vi "Read Sequential Addresses (CMD ONLY).vi"(7 "Target IC (1-8)":u8, 8 "error in (no error)":errorcluster, 9 "Addresses to Read":u16 format="%0.0f", 10 "Starting Address":u16 format="%04x", 11 "FPGA Interface in":refnum<class "FPGA Interface.lvclass">) -> (0 "error out":errorcluster)   [LabVIEW 2020, in "BCI-1553 API.lvlib" / "FPGA Interface.lvlib" / "FPGA Interface.lvclass"]
doc: "Reads a series of consecutive addresses from a component in the 1553 Session. Sequential addressing cannot be used on addresses from 0x0400 to 0x0800. This method does not block and will not wait for data to return from the specified component."
uses:
  FPGA Interface.lvclass
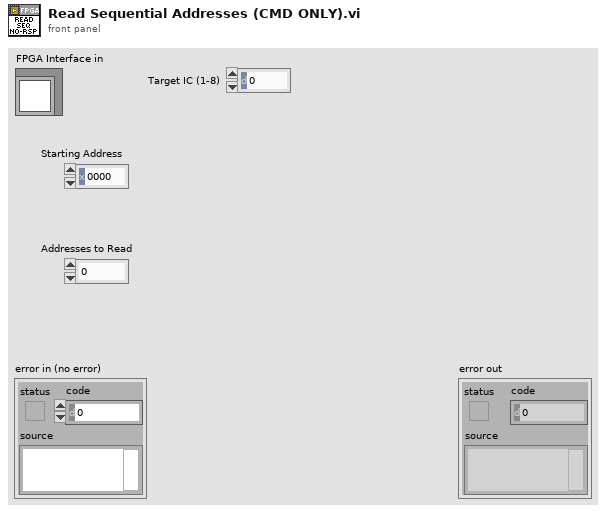
[diagram p1: front panel]
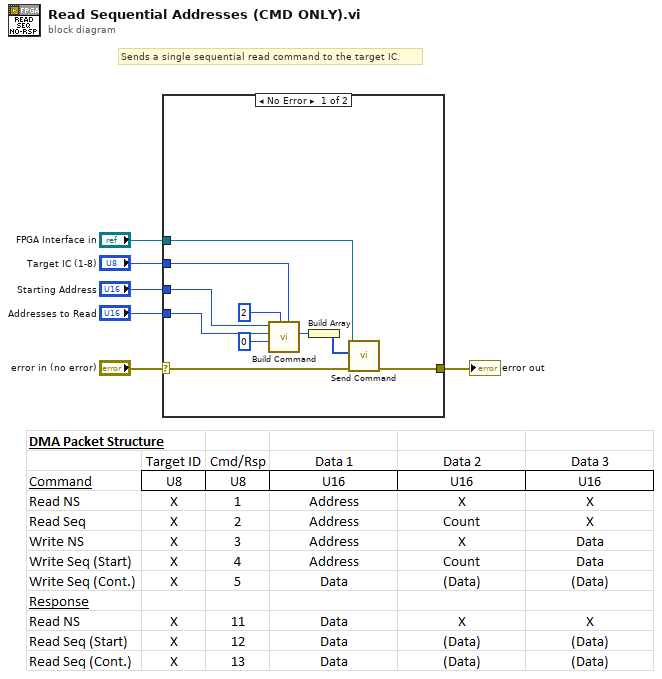
[diagram p0: block diagram]
diagram:
  # "Sends a single sequential read command to the target IC."
  n1 = case shown="No Error" "error in (no error)" {
    selector: "error in (no error)" -> [w13 w17]
    tunnel: [w7 w17] -> w5
    tunnel: "FPGA Interface in" -> [w11 _]
    tunnel: "Target IC (1-8)" -> [w12 _]
    tunnel: "Starting Address" -> [w10 _]
    tunnel: "Addresses to Read" -> [w8 _]
    frame No Error {
      n2 = call "Build Command.vi"("Target"=w12, "CMD ID"=u8 2, "Data 3"=u16 0, "Data 2"=w8, "Data 1"=w10) -> ("Command"=w16:u64)  [unwired: 5 in, 1 out]
      n3 = Build Array(w16) -> (w15:u64[])
      n4 = call "Send Command.vi"("error in (no error)"=w13, "Data"=w15, "FPGA Interface in"=w11) -> ("error out"=w7:errorcluster)  [unwired: 8 in]
    }
    frame Error {
    }
  }
  "error out" <- w5
